vi "UDP LA MOTOR Receive.vi"() -> ()   [LabVIEW 2017]
uses:
  Global 1.vi
panel:
  out "data out":string
  in  "Stop":bool
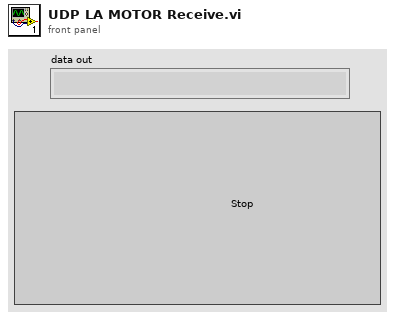
[diagram p1: front panel]
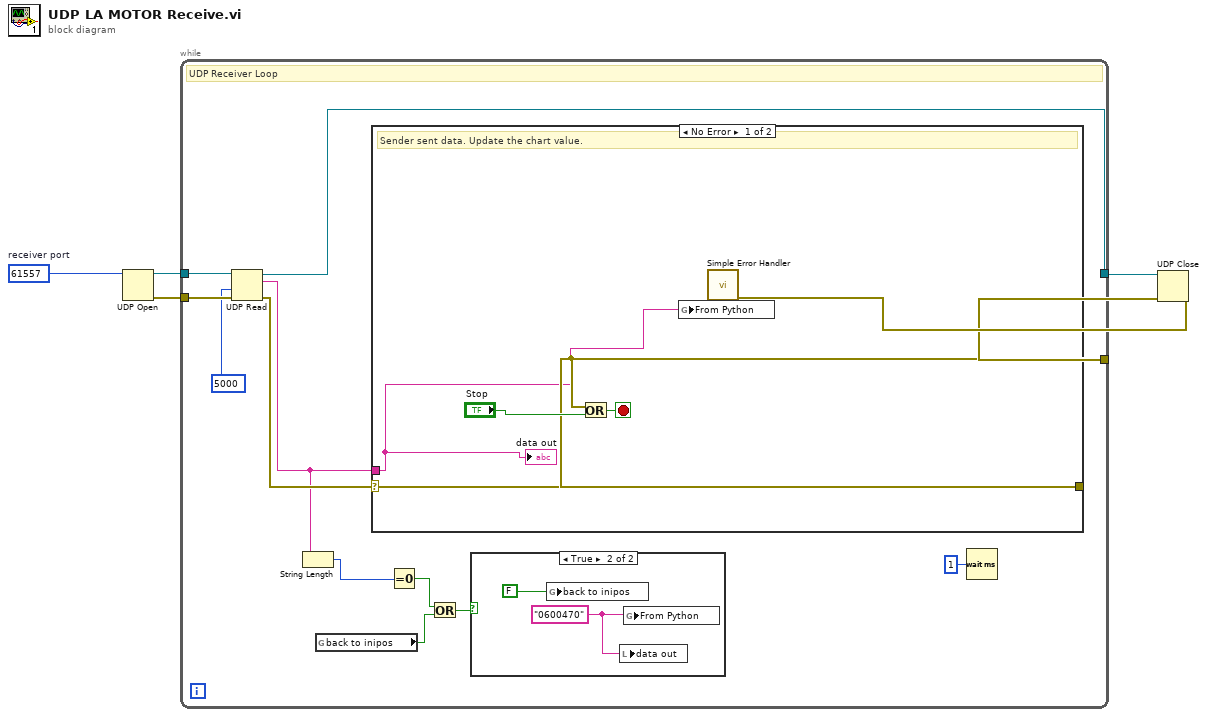
[diagram p0: block diagram]
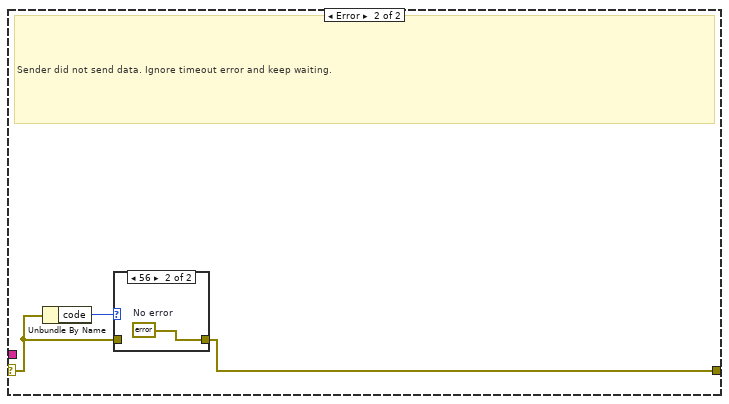
[diagram p3: hidden frame]
diagram:
  w1 = u16 61557  # receiver port
  n1 = UDP Open(11:w1) -> (port=w2:refnum<k16>, 0:w3:errorcluster)  [unwired: 4 in, 1 out]
  n2 = while {
    tunnel: w2 -> [w20]
    tunnel: [w13] -> w6
    tunnel: w3 -> [w17]
    tunnel: [w14] -> w4
    stop <- w18 stop-if-true
    # "UDP Receiver Loop"
    n3 = UDP Read(connection ID=w20, timeout ms (25000)=5000, 8:w17) -> (data out=w11:string, error out=w15:errorcluster, 3:w13:refnum<k16>)  [unwired: 3 out]
    n4 = String Length(string=w11) -> (length=w10:i32)
    n5 = global read "Global 1.vi" "back to inipos"() -> (w9:bool)
    n6 = case shown="No Error" w15 {
      selector: w15 -> [w24 w26]
      tunnel: w11 -> [w23 _]
      tunnel: [w24 w25] -> w14
      frame No Error {
        # "Sender sent data. Update the chart value."
        n7 = global write "Global 1.vi" "From Python"(w23) -> ()
        "data out" <- w23
      }
      frame Error {
        # "Sender did not send data. Ignore timeout error and keep waiting."
        n8 = Unbundle By Name(w26) -> ("code"=w27:i32)
        n9 = case shown="56" w27 {
          tunnel: w26 -> [w28 _]
          tunnel: [w28 w29] -> w25
          frame Default {
          }
          frame 56 {
            w29 = errorcluster {"status"=FALSE, "code"=0, "source"=""}  # No error
          }
        }
      }
    }
    n10 = Equal To 0?(x=w10) -> (x = 0?=w8:bool)
    n11 = Or(x=w8, y=w9) -> (x .or. y?=w7:bool)
    n12 = case shown="True" w7 {
      frame False {
      }
      frame True {
        w22 = "0600470" ("data out")
        n13 = global write "Global 1.vi" "back to inipos"(FALSE) -> ()
        n14 = local write "data out"(w22) -> ()
        n15 = global write "Global 1.vi" "From Python"(w22) -> ()
      }
    }
    n16 = Or(x=w14, y="Stop") -> (x .or. y?=w18:bool)
    n17 = Wait (ms)(milliseconds to wait=u32 1) -> ()  [unwired: 1 out]
  }
  n18 = UDP Close(connection ID=w6, 8:w4) -> (error out=w5:errorcluster)  [unwired: 1 out]
  n19 = call <vilib>:"Simple Error Handler.vi"("error in (no error)"=w5) -> ()  [unwired: 1 in, 8 out]
